vi "Add Events.vi"(8 "error in (no error)":errorcluster, 10 "Event Subs (All)":T1[](array[typedef]) items=["None"=0, "General"=1, "Config"=2, "Scenes"=4, "Inputs"=8, "Transitions"=16, "Filters"=32, "Outputs"=64, "SceneItems"=128, "MediaInputs"=256, "Vendors"=512, "UI"=1024, "NonHighVolume"=1023, "InputVolumeMeters"=65536, "InputActiveStateChanged"=131072, "InputShowStateChanged"=262144, "SceneItemTransformChanged"=524288], 11 "Identify in":refnum<class "Identify.lvclass">) -> (0 "error out":errorcluster, 3 "Identify out":refnum<class "Identify.lvclass">)   [LabVIEW 2020, in "obs-websocket.lvlib" / "Identify.lvclass"]
uses:
  Identify.lvclass
  Event Subscription.ctl
  Identify.lvclass/Identify.ctl
  obs-websocket.lvlib
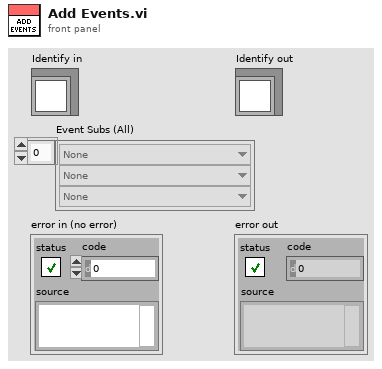
[diagram p1: front panel]
types:
  T1 = typedef "obs-websocket.lvlib/Event Subscription.ctl" = u32
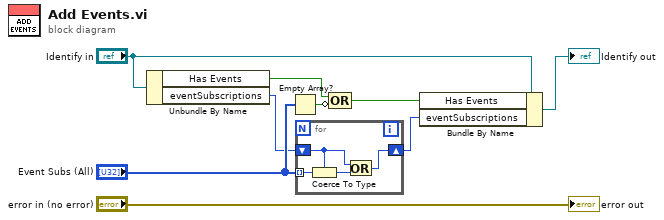
[diagram p0: block diagram]
diagram:
  n1 = Unbundle By Name("Identify in") -> ("Has Events"=w5:bool, "eventSubscriptions"=w4:u32)
  n2 = Empty Array?(array="Event Subs (All)") -> (empty?=w6:bool)
  n3 = for {
    tunnel: "Event Subs (All)" -> [w13] mode=indexing
    shift-right: [w10] -> w1
    shift-left: w4 -> [w11]
    n4 = Coerce To Type(0:w13, 1:w11) -> (2:w12:u32)
    n5 = Or(x=w11, y=w12) -> (x .or. y?=w10:u32)
  }
  n6 = Compound Arithmetic op=OR(w5, invert w6) -> (w2:bool)
  n7 = Bundle By Name(cluster="Identify in", "Has Events"=w2, "eventSubscriptions"=w1) -> (→"Identify out":refnum<class "Identify.lvclass">)
  "error out" <- "error in (no error)"
